vi "Error On Delimiter Found.vi"(7 "Delimiter":string, 8 "error in (no error)":errorcluster, 11 "Node Path":string) -> (0 "error out":errorcluster)   [LabVIEW 2020, in "Blue Tree Map OpenSource.lvlib"]
uses:
  Blue Tree Map OpenSource.lvlib
  <vilib>/Utility/error.llb/Error Cluster From Error Code.vi
  <vilib>/ErrorRing/Error Ring.xnode
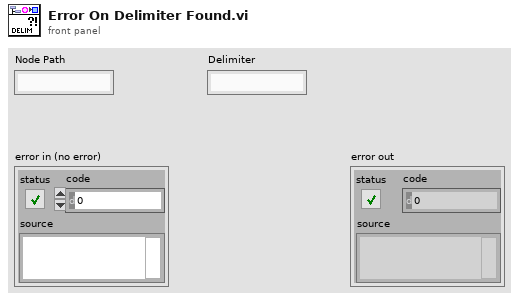
[diagram p1: front panel]
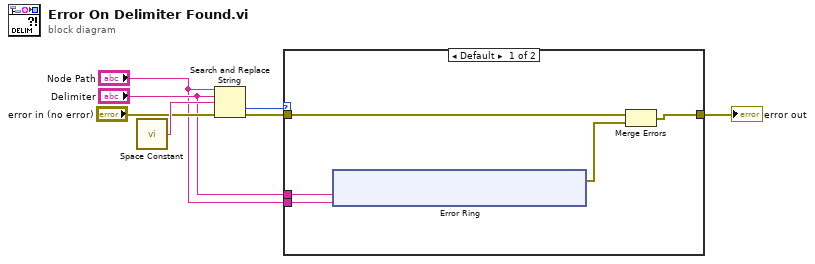
[diagram p0: block diagram]
diagram:
  n1 = call <vilib>:"Space Constant.vi"() -> ("String"=w7:string)
  n2 = Search and Replace String(input string="Node Path", search string="Delimiter", replace string=w7, error in="error in (no error)") -> (offset past replacement=w5:i32, error out=w4:errorcluster)  [unwired: 4 in, 2 out]
  n3 = case shown="Default" w5 {
    tunnel: w4 -> [w12 w21]
    tunnel: [w10 w21] -> w3
    tunnel: "Delimiter" -> [w9 _]
    tunnel: "Node Path" -> [w8 _]
    frame Default {
      n4 = xnode "Error Ring"("parameter 0"=w9, "parameter 1"=w8) -> ("error out"=w11:errorcluster)
      n5 = Merge Errors(w12, w11) -> (w10:errorcluster)
    }
    frame -1 {
    }
  }
  "error out" <- w3
